vi "Draw Glyph.vi"(5 "Transform (Center)":refnum<class "Transform.lvclass">, 6 "Colors":T1={"Front"={"Color"=0, "Alpha"=255}, "Back"={"Color"=16448250, "Alpha"=255}}, 7 "Font (System)":refnum<class "Font Settings.lvclass">, 8 "error in (no error)":errorcluster, 9 "Destination":refnum<class "Glyph Canvas.lvclass">, 10 "codepoint":u32, 11 "Glyph Drawer in":refnum<class "Glyph Drawer.lvclass">) -> (0 "error out":errorcluster, 1 "Destination Out":refnum<class "Glyph Canvas.lvclass">, 3 "Glyph Drawer out":refnum<class "Glyph Drawer.lvclass">)   [LabVIEW 2023, in "Font Glyph Drawer Interface.lvlib" / "Glyph Drawer.lvclass"]
uses:
  Glyph Drawer.lvclass
  Glyph Canvas/Glyph Canvas.lvclass
  Font Settings/Font Settings.lvclass
  Transform/Transform.lvclass
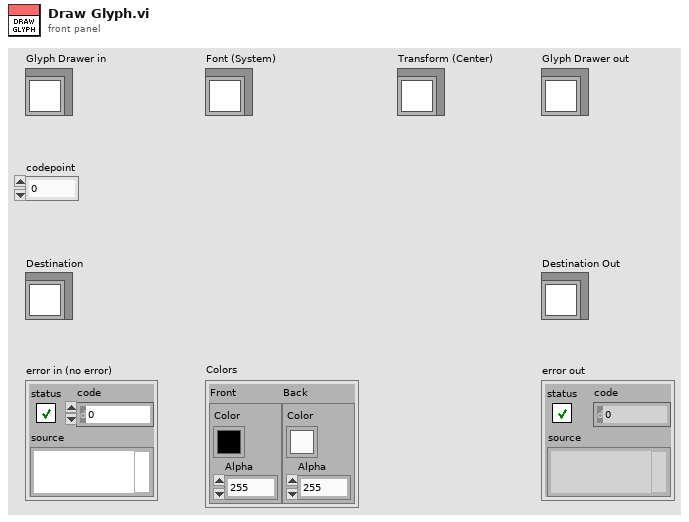
[diagram p1: front panel]
types:
  T1 = cluster{"Front":cluster{"Color":u32, "Alpha":u8}, "Back":cluster{"Color":u32, "Alpha":u8}}
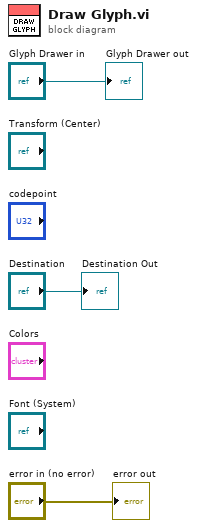
[diagram p0: block diagram]
diagram:
  "error out" <- "error in (no error)"
  "Glyph Drawer out" <- "Glyph Drawer in"
  "Destination Out" <- "Destination"
